vi "IMAQDevice.ProcEvents.vi"(0 "i ref in":refnum<vi>, 5 "error in (no error)":errorcluster) -> (14 "i ref out":refnum<vi>, 19 "error out":errorcluster)   [LabVIEW 2014, in "IMAQDevice.lvlib"]
doc: "This method is used to define the events the object will listen to. Add your own events here."
uses:
  IMAQDevice.lvlib
  CSCore/BaseProcess/BaseProcess.event definition.ctl
  CSCore/CAEObj/CAEObj.event definition.ctl
  CSCore/BaseProcess/BaseProcess.descriptor string definition.ctl
  CSCore/BaseProcess/BaseProcess.lvlib
  CSCore/CAEObj/CAEObj.lvlib
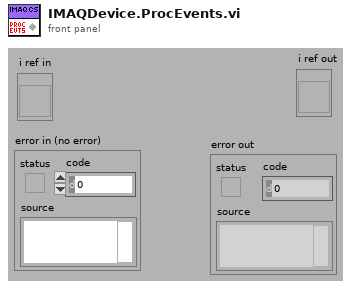
[diagram p1: front panel]
types:
  T1 = typedef "BaseProcess.lvlib/BaseProcess.event definition.ctl" = cluster{"CAEEvtDef":T2, "Data Descriptor":T3}
  T2 = typedef "CAEObj.lvlib/CAEObj.event definition.ctl" = cluster{"URL":string, "enable":bool, "ignoreResID":bool}
  T3 = typedef "BaseProcess.lvlib/BaseProcess.descriptor string definition.ctl" = string
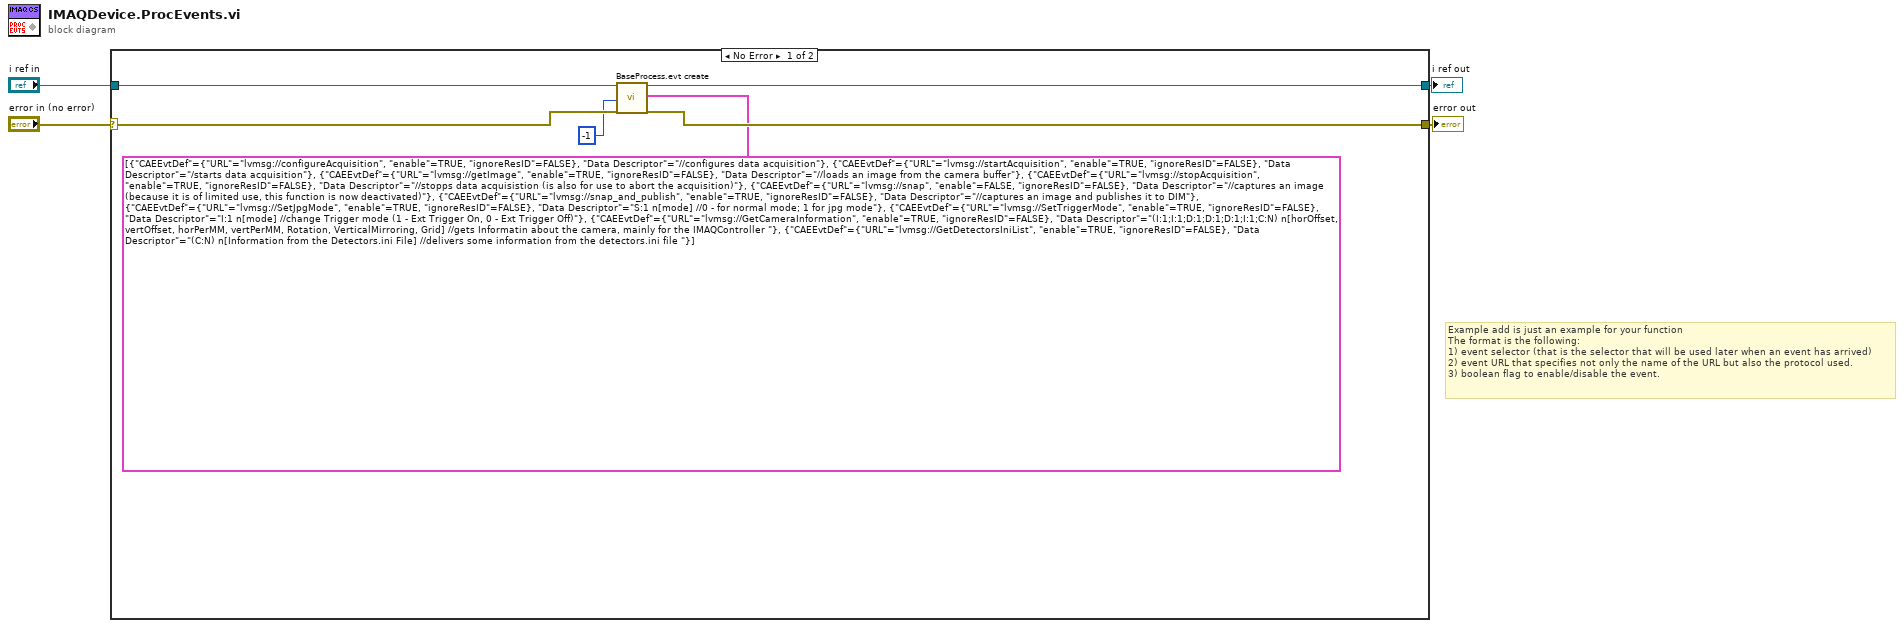
[diagram p0: block diagram]
diagram:
  # "Example add is just an example for your function\nThe format is the following:\n1) event selector (that is the selector that will be used later when an event has arrived)\n2) event URL that specifies not only the name of the URL but also the protocol used.\n3) boolean flag to enable/disable the event."
  n1 = case shown="No Error" "error in (no error)" {
    selector: "error in (no error)" -> [w6 w11]
    tunnel: "i ref in" -> [w10 w12]
    tunnel: [w9 w12] -> w3
    tunnel: [w8 w11] -> w2
    frame No Error {
      n2 = call "BaseProcess.evt create.vi"("i ref in"=w10, "newEvents"=T1[] [{"CAEEvtDef"={"URL"="lvmsg://configureAcquisition", "enable"=TRUE, "ignoreResID"=FALSE}, "Data Descriptor"="//configures data acquisition"}, {"CAEEvtDef"={"URL"="lvmsg://startAcquisition", "enable"=TRUE, "ignoreResID"=FALSE}, "Data Descriptor"="/starts data acquisition"}, {"CAEEvtDef"={"URL"="lvmsg://getImage", "enable"=TRUE, "ignoreResID"=FALSE}, "Data Descriptor"="//loads an image from the camera buffer"}, {"CAEEvtDef"={"URL"="lvmsg://stopAcquisition", "enable"=TRUE, "ignoreResID"=FALSE}, "Data Descriptor"="//stopps data acquisistion (is also for use to abort the acquisition)"}, {"CAEEvtDef"={"URL"="lvmsg://snap", "enable"=FALSE, "ignoreResID"=FALSE}, "Data Descriptor"="//captures an image (because it is of limited use, this function is now deactivated)"}, {"CAEEvtDef"={"URL"="lvmsg://snap_and_publish", "enable"=TRUE, "ignoreResID"=FALSE}, "Data Descriptor"="//captures an image and publishes it to DIM"}, {"CAEEvtDef"={"URL"="lvmsg://SetJpgMode", "enable"=TRUE, "ignoreResID"=FALSE}, "Data Descriptor"="S:1 n[mode] //0 - for normal mode; 1 for jpg mode"}, {"CAEEvtDef"={"URL"="lvmsg://SetTriggerMode", "enable"=TRUE, "ignoreResID"=FALSE}, "Data Descriptor"="I:1 n[mode] //change Trigger mode (1 - Ext Trigger On, 0 - Ext Trigger Off)"}, {"CAEEvtDef"={"URL"="lvmsg://GetCameraInformation", "enable"=TRUE, "ignoreResID"=FALSE}, "Data Descriptor"="(I:1;I:1;D:1;D:1;D:1;I:1;C:N) n[horOffset, vertOffset, horPerMM, vertPerMM, Rotation, VerticalMirroring, Grid] //gets Informatin about the camera, mainly for the IMAQController "}, {"CAEEvtDef"={"URL"="lvmsg://GetDetectorsIniList", "enable"=TRUE, "ignoreResID"=FALSE}, "Data Descriptor"="(C:N) n[Information from the Detectors.ini File] //delivers some information from the detectors.ini file "}] ("new events"), "ms timeout (10000)"=-1, "error in (no error)"=w6) -> ("i ref out"=w9:refnum<vi>, "error out"=w8:errorcluster)  [unwired: 12 in, 2 out]
    }
    frame Error {
    }
  }
  "i ref out" <- w3
  "error out" <- w2
